vi "Function_Generator.vi"(8 "error in (no error)":errorcluster, 9 "Simulated Input?":bool, 11 "Config Settings":T1) -> (0 "error out":errorcluster, 3 "Data Out":dbl[](array[numeric]))   [LabVIEW 2024]
uses:
  controls/Config_Settings.ctl
  <vilib>/measure/NI_MABase.lvlib
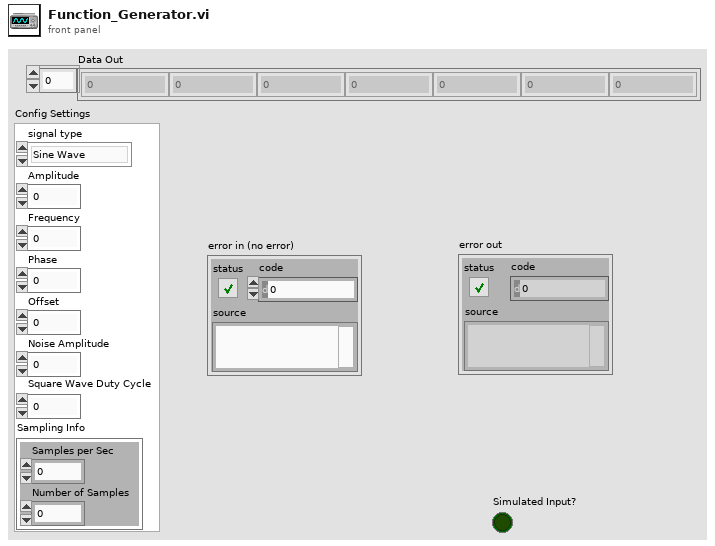
[diagram p1: front panel]
types:
  T1 = typedef "Config_Settings.ctl" = cluster{"signal type":enum16{"Sine Wave", "Triangle Wave", "Square Wave", "Sawtooth Wave"}, "Amplitude":dbl, "Frequency":dbl, "Phase":dbl, "Offset":dbl, "Noise Amplitude":dbl, "Square Wave Duty Cycle":dbl, "Sampling Info":cluster{"Samples per Sec":dbl, "Number of Samples":dbl}}
  T2 = enum16{"Sine Wave", "Triangle Wave", "Square Wave", "Sawtooth Wave"}
  T3 = cluster{"Samples per Sec":dbl, "Number of Samples":dbl}
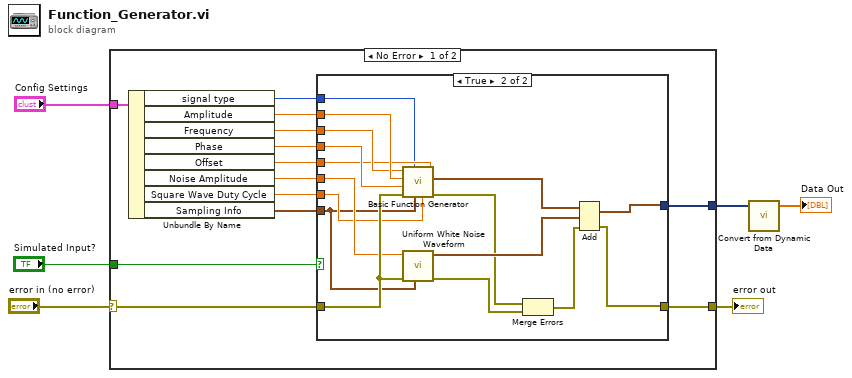
[diagram p0: block diagram]
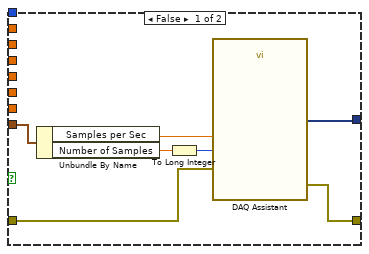
[diagram p2: hidden frame]
diagram:
  n1 = case shown="No Error" "error in (no error)" {
    selector: "error in (no error)" -> [w18 _]
    tunnel: [w19 _] -> w5
    tunnel: [w17 _] -> w4
    tunnel: "Config Settings" -> [w16 _]
    tunnel: "Simulated Input?" -> [w8 _]
    frame No Error {
      n2 = Unbundle By Name(w16) -> ("signal type"=w10:T2, "Amplitude"=w15:dbl, "Frequency"=w14:dbl, "Phase"=w13:dbl, "Offset"=w12:dbl, "Noise Amplitude"=w11:dbl, "Square Wave Duty Cycle"=w7:dbl, "Sampling Info"=w9:T3)
      n3 = case shown="True" w8 {
        tunnel: [w20 w40] -> w19
        tunnel: w18 -> [w21 w39]
        tunnel: [w26 w35] -> w17
        tunnel: w15 -> [_ w34]
        tunnel: w14 -> [_ w33]
        tunnel: w13 -> [_ w32]
        tunnel: w12 -> [_ w31]
        tunnel: w11 -> [_ w30]
        tunnel: w10 -> [_ w29]
        tunnel: w9 -> [w25 w27]
        tunnel: w7 -> [_ w28]
        frame False {
          n4 = Unbundle By Name(w25) -> ("Samples per Sec"=w24:dbl, "Number of Samples"=w23:dbl)
          n5 = To Long Integer(number=w23) -> (32bit integer=w22:i32)
          n6 = call "DAQ Assistant"("rate"=w24, "number of samples"=w22, "error in"=w21) -> ("data"=w26:dynamicdata, "error out"=w20:errorcluster)  [unwired: 14 in, 1 out]
        }
        frame True {
          n7 = call <vilib>:"Basic Function Generator.vi"("offset"=w31, "square wave duty cycle (%)"=w28, "sampling info"=w27, "signal type"=w29, "error in (no error)"=w39, "phase"=w32, "amplitude"=w34, "frequency"=w33) -> ("error out"=w37:errorcluster, "signal out"=w41:waveform(dbl))  [unwired: 1 in, 1 out]
          n8 = call <vilib>:"Uniform White Noise Waveform.vi"("sampling info"=w27, "error in (no error)"=w39, "amplitude"=w30) -> ("error out"=w36:errorcluster, "signal out"=w42:waveform(dbl))  [unwired: 7 in]
          n9 = Merge Errors(w37, w36) -> (w38:errorcluster)
          n10 = Add(1:w42, 2:w41, 4:w38) -> (0:w35:waveform(dbl), 3:w40:errorcluster)
        }
      }
    }
    frame Error {
    }
  }
  "error out" <- w5
  n11 = call "Convert from Dynamic Data"("Dynamic Data Type"=w4) -> ("Array"=→"Data Out":dbl[])  [unwired: 3 in]
